vi "Timetrace_meas_diag_realtime.vi"(6 "LD Signal":tag, 7 "Refresh in (s)":dbl, 8 "error in (no error)":errorcluster, 9 "Reference Signal":tag, 10 "Sensitivity":T1(ring), 11 "Max frequency (Hz)":dbl) -> (0 "error out":errorcluster, 1 "Sampling frequency":dbl, 2 "Number of samples":i16, 3 "Ref_MLD measurement":dbl[][](array[numeric]))   [LabVIEW 2013]
uses:
  <vilib>/DAQmx/read.llb/DAQmx Read (Analog 2D DBL NChan NSamp).vi
  <vilib>/DAQmx/create/channels.llb/DAQmx Create Channel (AI-Voltage-Basic).vi
  <vilib>/DAQmx/configure/timing.llb/DAQmx Timing (Sample Clock).vi
  <vilib>/DAQmx/miscellaneous.llb/DAQmx Fill In Error Info.vi
  <resource>/objmgr/daqmx.rc
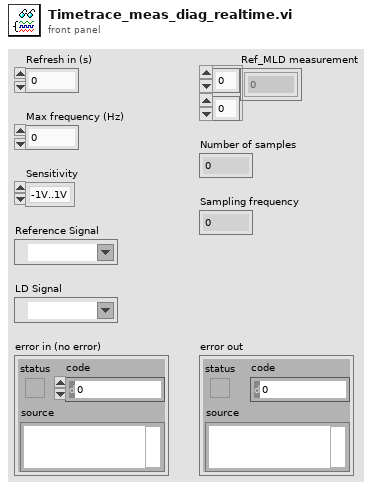
[diagram p1: front panel]
types:
  T1 = enum16{"-1V..1V", "-1.25V..1.25V", "-2V..2V", "-2.5V..2.5V", "-4V..4V", "-5V..5V", "-10V..10V"}
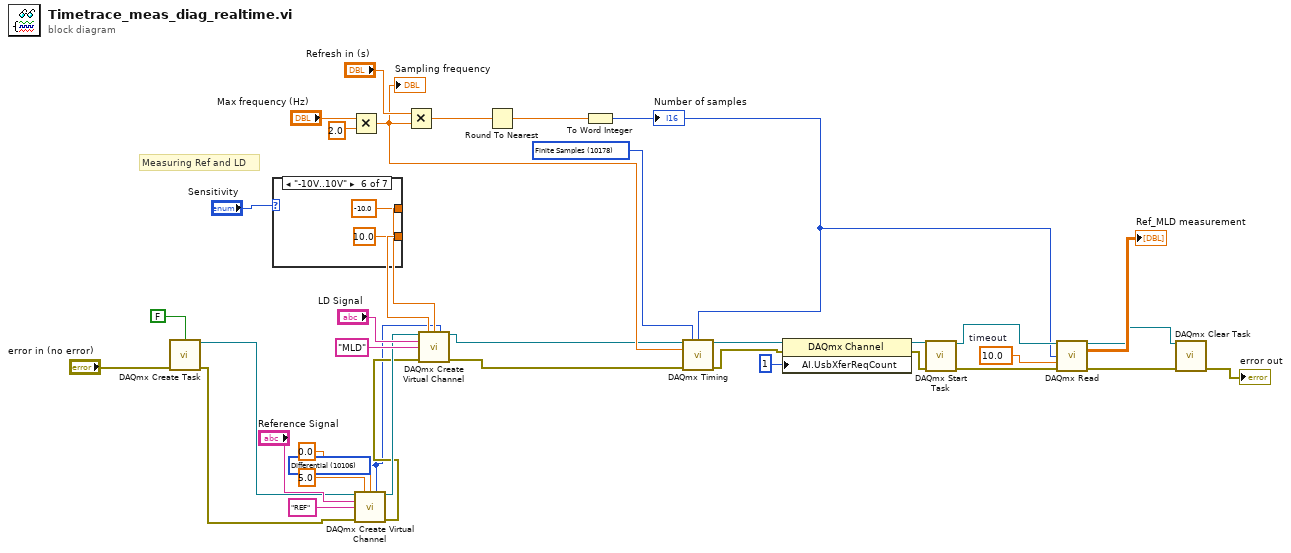
[diagram p0: block diagram]
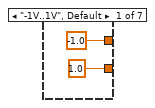
[diagram p2: hidden frame]
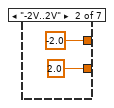
[diagram p3: hidden frame]
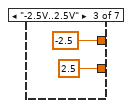
[diagram p4: hidden frame]
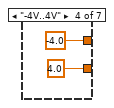
[diagram p5: hidden frame]
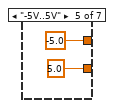
[diagram p6: hidden frame]
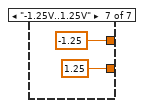
[diagram p7: hidden frame]
diagram:
  w1 = 10106 items=["default"=-1, "RSE"=10083, "NRSE"=10078, "Differential"=10106, "Pseudodifferential"=12529] ("input terminal configuration")
  w23 = 10.0  # timeout
  w21 = 10178 items=["Finite Samples"=10178, "Continuous Samples"=10123] ("sample mode")
  # "Measuring Ref and LD"
  n1 = call <vilib>:"DAQmx Create Task.vi"("auto cleanup"=FALSE, "error in"="error in (no error)") -> ("task out"=w7:refnum<k21>, "error out"=w6:errorcluster)  [unwired: 12 in]
  n2 = case shown="\"-10V..10V\"" "Sensitivity" {
    tunnel: [-1.0 -2.0 -2.5 -4.0 -5.0 -10.0 -1.25] -> w34
    tunnel: [1.0 2.0 2.5 4.0 5.0 10.0 1.25] -> w35
    frame "-1V..1V", Default {
    }
    frame "-2V..2V" {
    }
    frame "-2.5V..2.5V" {
    }
    frame "-4V..4V" {
    }
    frame "-5V..5V" {
    }
    frame "-10V..10V" {
    }
    frame "-1.25V..1.25V" {
    }
  }
  n3 = Multiply(x="Max frequency (Hz)", y=2.0) -> (x*y=w37:dbl)
  "Sampling frequency" <- w37
  n4 = call-poly <vilib>:"DAQmx Create Virtual Channel.vi"("task in"=w7, "maximum value"=5.0, "minimum value"=0.0, "input terminal configuration"=w1, "physical channels"="Reference Signal", "name to assign"="REF", "error in"=w6) -> ("task out"=w5:refnum<k21>, "error out"=w4:errorcluster)  [unwired: 7 in]
  n5 = Multiply(x="Refresh in (s)", y=w37) -> (x*y=w31:dbl)
  n6 = call-poly <vilib>:"DAQmx Create Virtual Channel.vi"("task in"=w5, "maximum value"=w35, "minimum value"=w34, "input terminal configuration"=w1, "physical channels"="LD Signal", "name to assign"="MLD", "error in"=w4) -> ("task out"=w3:refnum<k21>, "error out"=w2:errorcluster)  [unwired: 7 in]
  n7 = Round To Nearest(number=w31) -> (nearest integer value=w32:dbl)
  n8 = To Word Integer(number=w32) -> (16bit integer=w15:i16)
  "Number of samples" <- w15
  n9 = call-poly <vilib>:"DAQmx Timing.vi"("task/channels in"=w3, "sample mode"=w21, "samples per channel"=w15, "rate"=w37, "error in"=w2) -> ("task out"=w11:refnum<k21>, "error out"=w9:errorcluster)  [unwired: 9 in]
  n10 = property class="DAQmx Channel"(reference=w11, error in=w9, "AI.UsbXferReqCount"=u32 1) -> (reference out=w10:refnum<k21>, error out=w8:errorcluster)
  n11 = call <vilib>:"DAQmx Start Task.vi"("task/channels in"=w10, "error in"=w8) -> ("task out"=w19:refnum<k21>, "error out"=w18:errorcluster)  [unwired: 12 in]
  n12 = call-poly <vilib>:"DAQmx Read.vi"("task/channels in"=w19, "number of samples per channel"=w15, "timeout"=w23, "error in"=w18) -> ("task out"=w20:refnum<k21>, "data"=→"Ref_MLD measurement":dbl[][], "error out"=w22:errorcluster)  [unwired: 9 in]
  n13 = call <vilib>:"DAQmx Clear Task.vi"("task in"=w20, "error in"=w22) -> ("error out"=→"error out":errorcluster)  [unwired: 13 in]
